vi "Load Hot Pixel Map.vi"(8 "Error In":errorcluster, 9 "Verbose (F)":bool, 10 "Hot Pixel Map Target":T1, 11 "Hot Pixel Mask Image Path":path) -> (0 "Error Out":errorcluster, 3 "Mask Image Dimensions":i32[](array[numeric]))   [LabVIEW 2021, in "Image.lvlib"]
uses:
  Image.lvlib
  Image Hot Pixel Map Target.ctl
  <vilib>/Utility/error.llb/DialogType.ctl
  SwissSPAD/SwissSPAD Live_Image Display Options.ctl
  SwissSPAD/SwissSPAD Live_Settings List.ctl
  Notebook/Notebook.lvlib
  Arrays/Arrays.lvlib
  Error/Error.lvlib
  SwissSPAD/SwissSPAD Live.lvlib
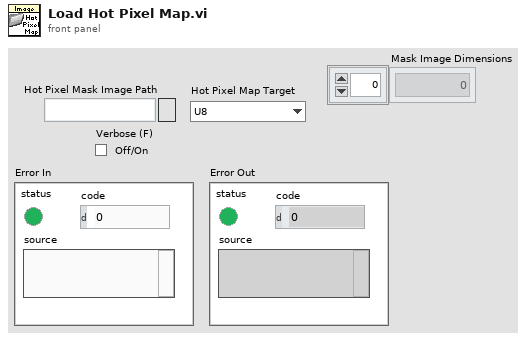
[diagram p1: front panel]
types:
  T1 = typedef "Image.lvlib/Image Hot Pixel Map Target.ctl" = enum16{"U8", "U16", "SGL"}
  T2 = typedef "SwissSPAD Live.lvlib/SwissSPAD Live_Settings List.ctl" = enum16{"FPGA:Bottom Half", "FPGA:Top Half", "FPGA:Bottom Bitfile Path", "FPGA:Top Bitfile Path", "FPGA:Bottom Bitstream Version", "FPGA:Top Bitstream Version", "FPGA:Auto Reset FPGA", "FPGA:Bottom FPGA Serial Number", "FPGA:Top FPGA Serial Number", "FPGA:Detector PCB Version", "Acquisition Parameters:Microlens", "Acquisition Parameters:SS2 DAQ Parameters", "Acquisition Parameters:Gate Configuration Array", "Acquisition Parameters:SS3 DAQ Parameters", "Acquisition Parameters:Buffer Size (# 8-bit Gates)", "File Information:File Information", "File Information:# Datasets in Series", "File Information:Scrambled File Flag", "File Information:SS3 Gate Slip Correction", "File Information:SS3 Hot Pixel Mismatch Detection", "File Information:Delay between Datasets", "File Information:Save Sum of All Gates Preview", "File Information:Preview Folder", "Image Parameters:Image ROI Information", "Image Parameters:Image Binning Options", "Image Parameters:SS3 Displayed Image", "Image Parameters:Image Display Options", "Image Parameters:Use Histogram Cursors", "Image Parameter:FPGA Data to Display", "UI Settings:Histogram Bins Number", "UI Settings:Histogram Bin Size", "UI Settings:Use Image Display Options", "UI Settings:Verbose Settings", "UI Settings:Verbose Saving"}
  T3 = typedef "SwissSPAD Live.lvlib/SwissSPAD Live_Image Display Options.ctl" = cluster{"Remove Screamers":bool, "Delta":sgl, "Equalize Histogram":bool, "Percentile":sgl, "Hot Pixel Mask Image":path, "Use Hot Pixel Mask":bool}
  T4 = typedef "Image Type" = u32
  T5 = typedef "IMAQ Image.ctl" = refnum<image>
  T6 = typedef "DialogType.ctl" = u16
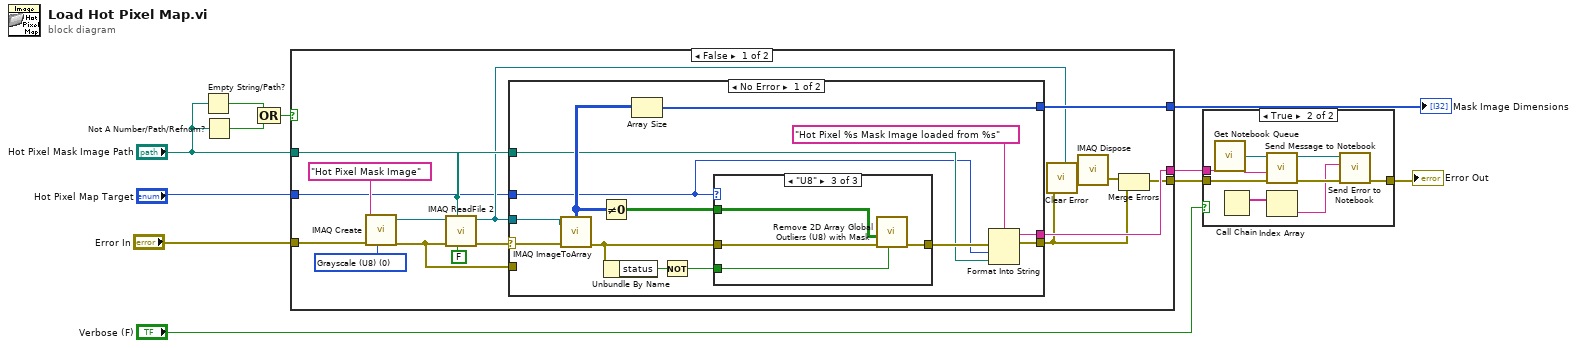
[diagram p0: block diagram]
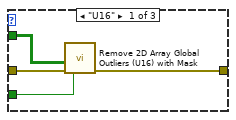
[diagram p3: hidden frame]
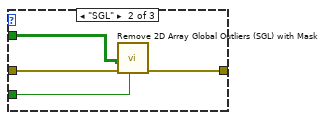
[diagram p4: hidden frame]
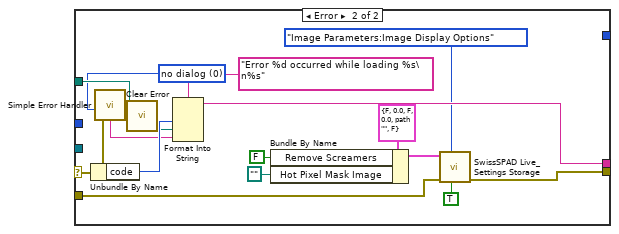
[diagram p5: hidden frame]
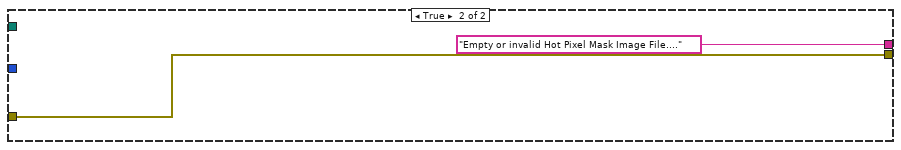
[diagram p6: hidden frame]
diagram:
  n1 = Empty String/Path?(string/path="Hot Pixel Mask Image Path") -> (empty?=w6:bool)
  n2 = Not A Number/Path/Refnum?(number/path/refnum="Hot Pixel Mask Image Path") -> (NaN/Path/Refnum?=w5:bool)
  n3 = Compound Arithmetic op=OR(w6, w5) -> (w4:bool)
  n4 = case shown="False" w4 {
    tunnel: "Error In" -> [w25 w71]
    tunnel: [w13 w71] -> w10
    tunnel: [w19 "Empty or invalid Hot Pixel Mask Image File...."] -> w9
    tunnel: "Hot Pixel Mask Image Path" -> [w20 _]
    tunnel: [w21 _] -> w3
    tunnel: "Hot Pixel Map Target" -> [w15 _]
    frame False {
      w26 = T4 0 items=["Grayscale (U8)", "Grayscale (I16)", "Grayscale (SGL)", "Complex (CSG)", "RGB (U32)", "HSL (U32)", "RGB (U64)", "Grayscale (U16)"] ("Image Type")
      n5 = call "IMAQ Create"("Image Name"="Hot Pixel Mask Image", "Image Type"=w26, "error in (no error)"=w25) -> ("New Image"=w24:T5, "error out"=w16:errorcluster)  [unwired: 2 in]
      n6 = call "IMAQ ReadFile 2"("Use File Path Image Type"=FALSE, "File Path"=w20, "error in (no error)"=w16, "Image"=w24) -> ("error out"=w22:errorcluster, "Image Out"=w17:T5)  [unwired: 3 in, 3 out]
      n7 = case shown="No Error" w22 {
        selector: w22 -> [w41 w65]
        tunnel: w17 -> [w38 _]
        tunnel: [w36 _] -> w21
        tunnel: [w30 w56] -> w12
        tunnel: w20 -> [w29 w68]
        tunnel: [w33 w67] -> w19
        tunnel: w16 -> [_ w57]
        tunnel: w15 -> [w28 _]
        frame No Error {
          n8 = call "IMAQ ImageToArray"("error in (no error)"=w41, "Image"=w38) -> ("error out"=w40:errorcluster, "Image Pixels (U8)"=w37:u8[][])  [unwired: 2 in, 3 out]
          n9 = Not Equal To 0?(x=w37) -> (x != 0?=w35:bool[][])
          n10 = Unbundle By Name(w40) -> ("status"=w39:bool)
          n11 = Array Size(array=w37) -> (size(s)=w36:i32[])
          n12 = Not(x=w39) -> (.not. x?=w34:bool)
          n13 = case shown="\"U8\"" w28 {
            tunnel: w40 -> [w45 w47 w50]
            tunnel: w35 -> [w44 w49 w53]
            tunnel: w34 -> [w43 w48 w52]
            tunnel: [w42 w46 w51] -> w32
            frame "U16" {
              n14 = call "Remove 2D Array Global Outliers (U16) with Mask.vi"("Init?"=w43, "Error In"=w45, "2D Mask in"=w44) -> ("Error Out"=w42:errorcluster)  [unwired: 5 in, 3 out]
            }
            frame "SGL" {
              n15 = call "Remove 2D Array Global Outliers (SGL) with Mask.vi"("Init?"=w48, "Error In"=w47, "2D Mask in"=w49) -> ("Error Out"=w46:errorcluster)  [unwired: 6 in, 2 out]
            }
            frame "U8" {
              n16 = call "Remove 2D Array Global Outliers (U8) with Mask.vi"("Init?"=w52, "Error In"=w50, "2D Mask in"=w53) -> ("Error Out"=w51:errorcluster)  [unwired: 5 in, 3 out]
            }
          }
          n17 = Format Into String(format string="Hot Pixel %s Mask Image loaded from %s", error in=w32, w28, w29) -> (resulting string=w33:string, error out=w30:errorcluster)  [unwired: 1 in]
        }
        frame Error {
          w62 = T6 0 items=["no dialog", "OK message", "continue or stop message", "OK message + warnings", "continue/stop + warnings"] ("type of dialog (OK msg:1)")
          n18 = Unbundle By Name(w65) -> ("code"=w69:i32)
          n19 = call <vilib>:"Simple Error Handler.vi"("type of dialog (OK msg:1)"=w62, "error in (no error)"=w65) -> ("error out"=w63:errorcluster, "message"=w64:string)  [unwired: 3 in, 3 out]
          n20 = call "Clear Error.vi"("Error In"=w63) -> ()  [unwired: 8 in, 1 out]
          n21 = Format Into String(format string="Error %d occurred while loading %s\n%s", w69, w68, w64) -> (resulting string=w67:string)  [unwired: 2 in, 1 out]
          n22 = Bundle By Name(cluster=T3 {"Remove Screamers"=FALSE, "Delta"=0.0, "Equalize Histogram"=FALSE, "Percentile"=0.0, "Hot Pixel Mask Image"=path "", "Use Hot Pixel Mask"=FALSE} ("Image Display Options"), "Remove Screamers"=FALSE, "Hot Pixel Mask Image"=path "") -> (w61:T3)
          n23 = call "SwissSPAD Live_Settings Storage.vi"("Set/Get(F)"=TRUE, "Settings List"=SwissSPAD_Live_Settings_List."Image Parameters:Image Display Options", "Error In"=w57, "Variant Data in"=w61) -> ("Error Out"=w56:errorcluster)  [unwired: 6 in, 1 out]
        }
      }
      n24 = call "Clear Error.vi"("Error In"=w12) -> ("no Error Out"=w14:errorcluster)  [unwired: 8 in]
      n25 = call "IMAQ Dispose"("Image"=w17, "error in (no error)"=w14) -> ("error out"=w18:errorcluster)  [unwired: 4 in]
      n26 = Merge Errors(w18, w12) -> (w13:errorcluster)
    }
    frame True {
    }
  }
  "Mask Image Dimensions" <- w3
  n27 = case shown="True" "Verbose (F)" {
    tunnel: w10 -> [w72 w80]
    tunnel: w9 -> [_ w79]
    tunnel: [w72 w76] -> w8
    frame False {
    }
    frame True {
      n28 = call "Get Notebook Queue.vi"() -> ("Notebook Queue"=w78:refnum<queue>)  [unwired: 9 in]
      n29 = Call Chain() -> (call chain=w74:string[])
      n30 = call "Send Message to Notebook.vi"("Error In"=w80, "Message"=w79, "Notebook Queue"=w78) -> ("Error Out"=w77:errorcluster, "Notebook Queue"=w75:refnum<queue>)  [unwired: 5 in]
      n31 = Index Array(array=w74) -> (element=w73:string)  [unwired: 1 in]
      n32 = call "Send Error to Notebook.vi"("error in (no error)"=w77, "State Machine Case Error Source"=w73, "Notebook Q"=w75) -> ("Error Out"=w76:errorcluster)  [unwired: 8 in]
    }
  }
  "Error Out" <- w8
